vi "GetDistance2TL.vi"(3 "Traffic Lights":T1, 4 "Truck Dimensions":dbl[](array[numeric]), 5 "Trajectory Network":T2(array[cluster]), 6 "CurrentWP":i32[](array[numeric]), 7 "Trucks Poses":dbl[][](array[numeric]), 8 "Current State":i32[](array[numeric])=[1, 1, 1]) -> (0 "StopArray_2":i32[](array[numeric]), 1 "d2TLFinal":dbl[](array[numeric]), 2 "StopArray_1":i32[](array[numeric]))   [LabVIEW 2013]
uses:
  <vilib>/imath/engines/lvmath/Plug In/_Char/NIMS_CH_character datatype.ctl
  <vilib>/imath/engines/lvmath2/RunTimeEngine/ErrorHandling/NIMS_Finalize Error.vi
  <vilib>/imath/engines/lvmath2/RunTimeEngine/Managers/WorkSpace/UID Generator.vi
  <vilib>/imath/engines/lvmath2/RunTimeEngine/BuiltInFunctions/size/NIMS_I32=size(GM,I32).vi
  <instcachedir>/0/NIMS_I32=size(GM,I32)_0501686D1A7F4581B546512A0CE6115B.lvgen/NIMS_I32=size(GM,I32)_0501686D1A7F4581B546512A0CE6115B_004.vi
  <vilib>/imath/engines/lvmath2/RunTimeEngine/BuiltInFunctions/zeros/NIMS_M=zeros(I32,I32).vi
  <vilib>/imath/engines/lvmath2/RunTimeEngine/ErrorHandling/NIMS_Create Error From Enums.vi
  <vilib>/imath/engines/lvmath2/RunTimeEngine/BuiltInFunctions/ones/NIMS_M=ones(I32,I32).vi
  <vilib>/imath/engines/lvmath2/RunTimeEngine/BuiltInFunctions/zeros/NIMS_V=zeros(I32,I32).vi
  <vilib>/imath/engines/lvmath2/RunTimeEngine/RangeToken/NIMS_Range_R2 - Integer.vi
  <instcachedir>/0/NIMS_Range_R2 - Integer_C51C130E5EA5464EA148B28CDAB9615A.lvgen/NIMS_Range_R2 - Integer_C51C130E5EA5464EA148B28CDAB9615A_000.vi
  <vilib>/imathl/engines/lvmath/Functions/Error Handling/Create Error.vi
  <vilib>/imath/engines/lvmath2/RunTimeEngine/Managers/SymbolTable/Clear UID.vi
  <vilib>/imath/engines/lvmath2/RunTimeEngine/NodeEndStatement/NIMS_NodeEndStatement_Output.vi
  <instcachedir>/0/NIMS_NodeEndStatement_Output_53EC0D466D134D7ABD903AC30B43404B.lvgen/NIMS_NodeEndStatement_Output_53EC0D466D134D7ABD903AC30B43404B_004.vi
  <instcachedir>/0/NIMS_NodeEndStatement_Output_53EC0D466D134D7ABD903AC30B43404B.lvgen/NIMS_NodeEndStatement_Output_53EC0D466D134D7ABD903AC30B43404B_000.vi
  <vilib>/imath/engines/lvmath2/RunTimeEngine/CommandStatement/MC_CommandStatement_break.vi
  <vilib>/imath/engines/lvmath2/RunTimeEngine/IndexRead/NIMS V(S).vi
  <instcachedir>/0/NIMS V(S)_0488751826AF41519A22953C041130DC.lvgen/NIMS V(S)_0488751826AF41519A22953C041130DC_002.vi
  <vilib>/imath/engines/lvmath2/RunTimeEngine/IndexRead/NIMS M(S,S).vi
  <instcachedir>/0/NIMS M(S,S)_AC51E74150A542F7991B9634C66F3096.lvgen/NIMS M(S,S)_AC51E74150A542F7991B9634C66F3096_000.vi
  <vilib>/imath/engines/lvmath2/RunTimeEngine/BuiltInFunctions/deg_to_rad/NIMS_deg_to_rad.vi
  <instcachedir>/0/NIMS_deg_to_rad_4A81D684CE8D4DD79924F5AB74D756E1.lvgen/NIMS_deg_to_rad_4A81D684CE8D4DD79924F5AB74D756E1_001.vi
  <vilib>/imath/engines/lvmath2/RunTimeEngine/BuiltInFunctions/atan2/NIMS_atan2.vi
  <instcachedir>/0/NIMS_atan2_A91AA4A7D42247EDBE8F76DB99AF04A4.lvgen/NIMS_atan2_A91AA4A7D42247EDBE8F76DB99AF04A4_000.vi
  <vilib>/imath/engines/lvmath/Plug In/_Char/NIMS_CH_Character RV to String.vi
  <vilib>/imath/engines/lvmath2/RunTimeEngine/BuiltInFunctions/fprintf/NIMS_fprintf(Str,RS,RS).vi
  <vilib>/imath/engines/lvmath2/RunTimeEngine/IndexReplace/NIMS M(S,S)=S.vi
  <instcachedir>/0/NIMS M(S,S)=S_EC2A86BD47664E68AE45685B0A86CA9E.lvgen/NIMS M(S,S)=S_EC2A86BD47664E68AE45685B0A86CA9E_001.vi
  <vilib>/imath/engines/lvmath2/RunTimeEngine/RunTimeType/NIMS_RunTimeType_From StrictType (excl LVString).vi
  <instcachedir>/0/NIMS_RunTimeType_From StrictType (excl LVString)_4DEE718D6EB74582AA20236969C084FC.lvgen/NIMS_RunTimeType_From StrictType (excl LVString)_4DEE718D6EB74582AA20236969C084FC_000.vi
  <vilib>/imath/engines/lvmath2/RunTimeEngine/LocalVariableDefStatement/MC_LocalVariableDefStatement_Display.vi
  <vilib>/imath/engines/lvmath2/RunTimeEngine/IndexRead/NIMS M(S,$).vi
  <instcachedir>/0/NIMS M(S,$)_F24F360562DE41D8BE234322A2E15C65.lvgen/NIMS M(S,$)_F24F360562DE41D8BE234322A2E15C65_001.vi
  <vilib>/imath/engines/lvmath2/RunTimeEngine/BuiltInFunctions/sort/NIMS_sort(CRowV,I32,Str).vi
  <instcachedir>/0/NIMS_sort(CRowV,I32,Str)_29346373CFC04663A860DA4419001647.lvgen/NIMS_sort(CRowV,I32,Str)_29346373CFC04663A860DA4419001647_000.vi
  <vilib>/imath/engines/lvmath2/RunTimeEngine/BuiltInFunctions/findnz/NIMS_[1o]_findnz(GRowV).vi
  <instcachedir>/0/NIMS_[1o]_findnz(GRowV)_A907680C39E74AF18CBD76E991AC1137.lvgen/NIMS_[1o]_findnz(GRowV)_A907680C39E74AF18CBD76E991AC1137_000.vi
  <vilib>/imath/engines/lvmath2/RunTimeEngine/BuiltInFunctions/length/NIMS_length(GV).vi
  <instcachedir>/0/NIMS_length(GV)_08A3D13377FD4E4B96F5795FBF3698FA.lvgen/NIMS_length(GV)_08A3D13377FD4E4B96F5795FBF3698FA_002.vi
  <vilib>/imath/engines/lvmath2/RunTimeEngine/VariableToken/Support/NIMS_Vector Boolean Index to I32 Index.vi
  <vilib>/imath/engines/lvmath2/RunTimeEngine/IndexReplace/NIMS V(V)=M.vi
  <instcachedir>/0/NIMS V(V)=M_3D179AF5652E4922BC7E7B3B6BD740B2.lvgen/NIMS V(V)=M_3D179AF5652E4922BC7E7B3B6BD740B2_000.vi
  <instcachedir>/0/NIMS V(S)_0488751826AF41519A22953C041130DC.lvgen/NIMS V(S)_0488751826AF41519A22953C041130DC_005.vi
  <vilib>/imath/engines/lvmath2/RunTimeEngine/IndexReplace/NIMS V(S)=S.vi
  <instcachedir>/0/NIMS V(S)=S_66A18068148B4981A312229A93EA5C06.lvgen/NIMS V(S)=S_66A18068148B4981A312229A93EA5C06_001.vi
  <vilib>/imath/engines/lvmath2/RunTimeEngine/IndexRead/NIMS V(R2).vi
  <instcachedir>/0/NIMS V(R2)_C76619605A0E4E9F8B2FA9389712AC47.lvgen/NIMS V(R2)_C76619605A0E4E9F8B2FA9389712AC47_002.vi
  <vilib>/imath/engines/lvmath2/RunTimeEngine/IndexRead/NIMS V(V).vi
  <instcachedir>/0/NIMS V(V)_298D9CB7BFEB42B8BC8D9C3C28AE8C70.lvgen/NIMS V(V)_298D9CB7BFEB42B8BC8D9C3C28AE8C70_002.vi
  <vilib>/imath/engines/lvmath2/RunTimeEngine/BuiltInFunctions/sum/NIMS_sum(GV).vi
  <instcachedir>/0/NIMS_sum(GV)_67F5EC36BC034E54A6BEC5B0673C00E5.lvgen/NIMS_sum(GV)_67F5EC36BC034E54A6BEC5B0673C00E5_000.vi
  <vilib>/imath/engines/lvmath2/RunTimeEngine/Managers/SymbolTable/NIMS_WorkSpace.lvlib
panel:
  out "StopArray_2_before":i32[](array[numeric])
  out "d2TL_1":dbl[](array[numeric])
  out "d2TL_2":dbl[](array[numeric])
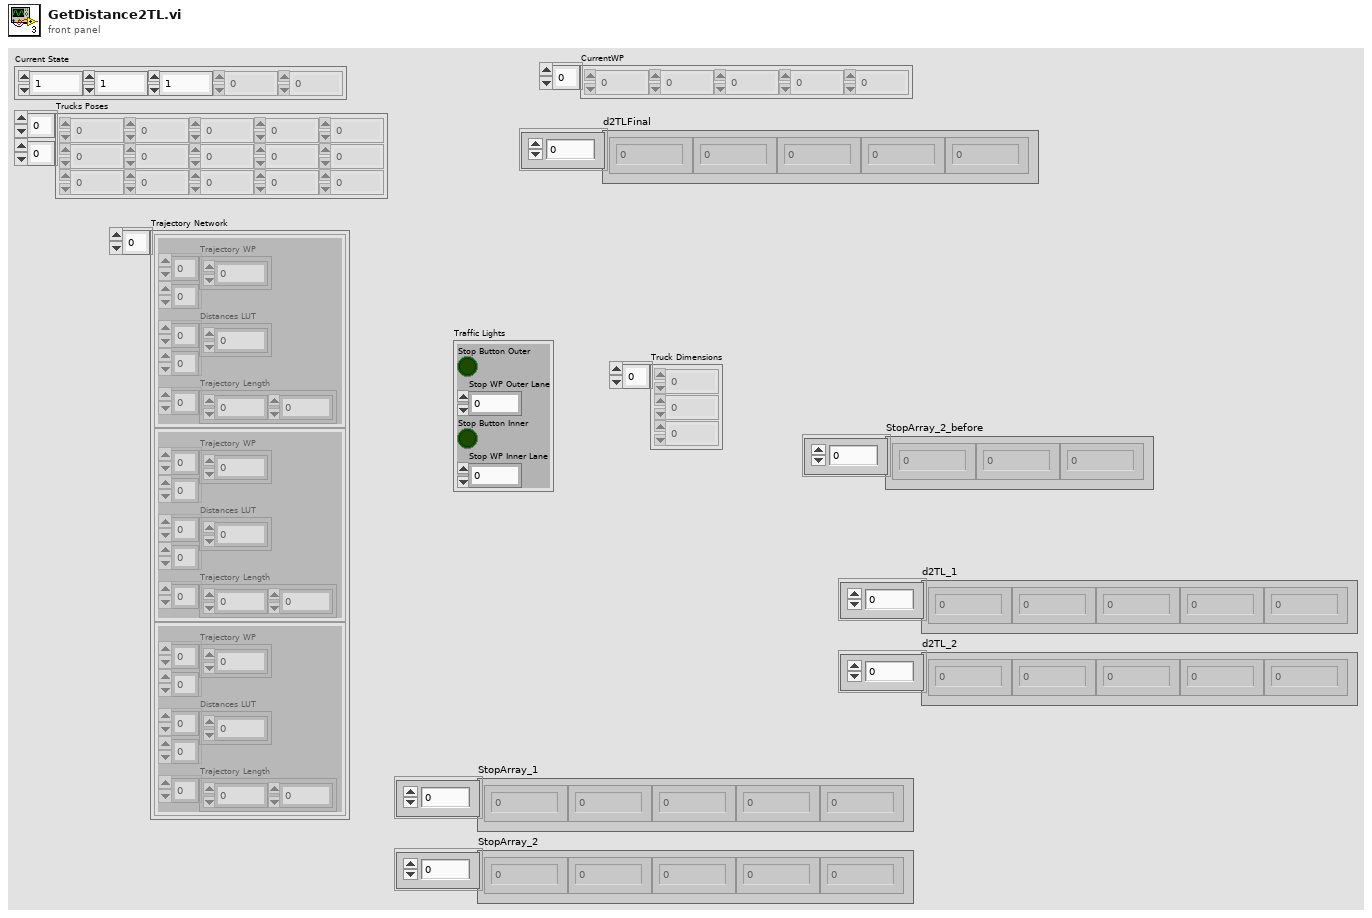
[diagram p1: front panel]
types:
  T1 = cluster{"Stop Button Outer":bool, "Stop WP Outer Lane":i32, "Stop Button Inner":bool, "Stop WP Inner Lane ":i32}
  T2 = cluster{"Trajectory WP":dbl[][], "Distances LUT":dbl[][], "Trajectory Length":i32[]}[]
  T3 = cluster{"Trajectory WP":dbl[][], "Distances LUT":dbl[][], "Trajectory Length":i32[]}
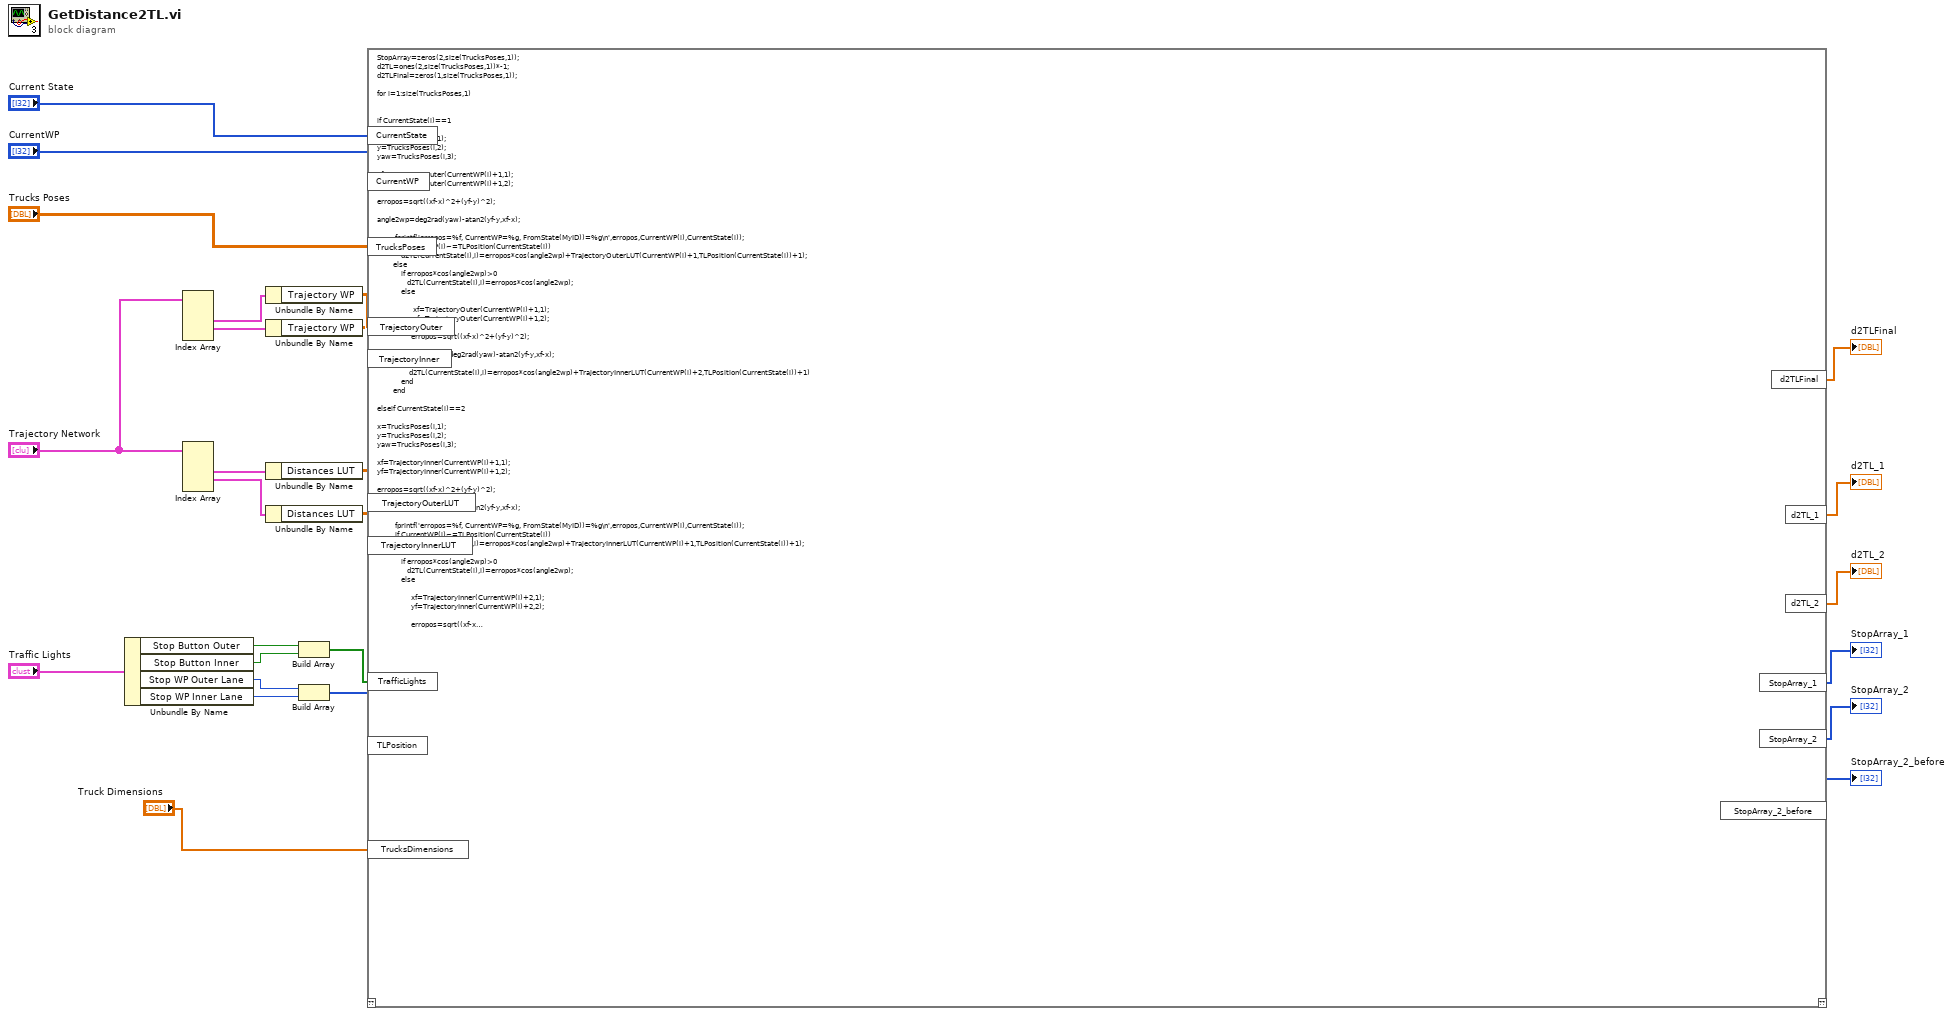
[diagram p0: block diagram]
diagram:
  n1 = Unbundle By Name("Traffic Lights") -> ("Stop Button Outer"=w15:bool, "Stop Button Inner"=w14:bool, "Stop WP Outer Lane"=w12:i32, "Stop WP Inner Lane"=w13:i32)
  n2 = Index Array(array="Trajectory Network") -> (element #2=w24:T3, element #3=w25:T3)  [unwired: 4 in, 2 out]
  n3 = Index Array(array="Trajectory Network") -> (element #2=w21:T3, element #3=w20:T3)  [unwired: 4 in, 2 out]
  n4 = Unbundle By Name(w24) -> ("Trajectory WP"=w23:dbl[][])
  n5 = Unbundle By Name(w25) -> ("Trajectory WP"=w22:dbl[][])
  n6 = Unbundle By Name(w21) -> ("Distances LUT"=w18:dbl[][])
  n7 = Unbundle By Name(w20) -> ("Distances LUT"=w17:dbl[][])
  n8 = Build Array(w15, w14) -> (w11:bool[])
  n9 = Build Array(w12, w13) -> (w10:i32[])
  n10 = mathscript code="StopArray=zeros(2,size(TrucksPoses,1));\nd2TL=ones(2,size(TrucksPoses,1))*-1;\nd2TLFinal=zeros(1,size(TrucksPoses,1));\n\nfor i=1:size(TrucksPoses,1)\n\n\nif CurrentState(i)==1\n\nx=TrucksPoses(i,1);\ny=TrucksPoses(i,2);\nyaw=TrucksPoses(i,3);\n\nxf=TrajectoryOuter(CurrentWP(i)+1,1);\nyf=TrajectoryOuter(CurrentWP(i)+1,2);\n\nerropos=sqrt((xf-x)^2+(yf-y)^2);\n\nangle2wp=deg2rad(yaw)-atan2(yf-y,xf-x);\n\n         fprintf('erropos=%f, CurrentWP=%g, FromState(MyID))=%g\\n',erropos,CurrentWP(i),CurrentState(i));\n         if CurrentWP(i)~=TLPosition(CurrentState(i))\n            d2TL(CurrentState(i),i)=erropos*cos(angle2wp)+TrajectoryOuterLUT(CurrentWP(i)+1,TLPosition(CurrentState(i))+1);\n        else\n            if erropos*cos(angle2wp)>0\n               d2TL(CurrentState(i),i)=erropos*cos(angle2wp);\n            else\n\n                  xf=TrajectoryOuter(CurrentWP(i)+1,1);\n                  yf=TrajectoryOuter(CurrentWP(i)+1,2);\n\n                 erropos=sqrt((xf-x)^2+(yf-y)^2);\n\n                 angle2wp=deg2rad(yaw)-atan2(yf-y,xf-x);\n                \n                d2TL(CurrentState(i),i)=erropos*cos(angle2wp)+TrajectoryInnerLUT(CurrentWP(i)+2,TLPosition(CurrentState(i))+1)\n            end\n        end\n\nelseif CurrentState(i)==2\n\nx=TrucksPoses(i,1);\ny=TrucksPoses(i,2);\nyaw=TrucksPoses(i,3);\n\nxf=TrajectoryInner(CurrentWP(i)+1,1);\nyf=TrajectoryInner(CurrentWP(i)+1,2);\n\nerropos=sqrt((xf-x)^2+(yf-y)^2);\n\nangle2wp=deg2rad(yaw)-atan2(yf-y,xf-x);\n\n         fprintf('erropos=%f, CurrentWP=%g, FromState(MyID))=%g\\n',erropos,CurrentWP(i),CurrentState(i));\n         if CurrentWP(i)~=TLPosition(CurrentState(i))\n            d2TL(CurrentState(i),i)=erropos*cos(angle2wp)+TrajectoryInnerLUT(CurrentWP(i)+1,TLPosition(CurrentState(i))+1);\n        else\n            if erropos*cos(angle2wp)>0\n               d2TL(CurrentState(i),i)=erropos*cos(angle2wp);\n            else\n\n                 xf=TrajectoryInner(CurrentWP(i)+2,1);\n                 yf=TrajectoryInner(CurrentWP(i)+2,2);\n\n                 erropos=sqrt((xf-x)^2+(yf-y)^2);\n\n                 angle2wp=deg2rad(yaw)-atan2(yf-y,xf-x);\n                \n                d2TL(CurrentState(i),i)=erropos*cos(angle2wp)+TrajectoryInnerLUT(CurrentWP(i)+2,TLPosition(CurrentState(i))+1)\n            end\n        end\n\nend\n\nend\n\nd2TL_1=d2TL(1,:);\nd2TL_2=d2TL(2,:);\n\n\n[spare, StopArray_1]=sort(d2TL_1);\n[spare, StopArray_2]=sort(d2TL_2);\n\nStopArray_2_before=StopArray_2;\n\nf1=find(d2TL_1==-1);\nf2=find(d2TL_2==-1)\n\nif length(f1)>0\n    for i=1:length(f1)\n        StopArray_1(StopArray_1==f1(i))=[];\n    end\nend\nif length(f2)>0\n    for i=1:length(f2)\n        StopArray_2(StopArray_2==f2(i))=[];\n    end\nend\n\ndref2TL=0.3;\n\nif length(StopArray_1)>0\n    d2TLFinal(StopArray_1(1))=d2TL_1(StopArray_1(1));\n    for i=2:length(StopArray_1)\n        d2TLFinal(StopArray_1(i))=d2TL_1(StopArray_1(i))-sum(TrucksDimensions(StopArray_1(1:i-1)))-dref2TL*(i-1);\n    end\nend\n\nif length(StopArray_2)>0\n    d2TLFinal(StopArray_2(1))=d2TL_2(StopArray_2(1));\n    for i=2:length(StopArray_2)\n        d2TLFinal(StopArray_2(i))=d2TL_2(StopArray_2(i))-sum(TrucksDimensions(StopArray_2(1:i-1)))-dref2TL*(i-1);\n    end\nend\n\nStopArray_1=[StopArray_1,zeros(1,size(TrucksPoses,1)-length(StopArray_1))];\nStopArray_2=[StopArray_2,zeros(1,size(TrucksPoses,1)-length(StopArray_2))];"("CurrentState"="Current State", "CurrentWP"="CurrentWP", "TrucksPoses"="Trucks Poses", "TrafficLights"=w11, "TrajectoryOuterLUT"=w18, "TLPosition"=w10, "TrajectoryInner"=w22, "TrajectoryOuter"=w23, "TrajectoryInnerLUT"=w17, "TrucksDimensions"="Truck Dimensions") -> ("d2TLFinal"=→"d2TLFinal":cdb[], "d2TL_1"=→"d2TL_1":cdb[], "d2TL_2"=→"d2TL_2":cdb[], "StopArray_1"=→"StopArray_1":i32[], "StopArray_2"=→"StopArray_2":i32[], "StopArray_2_before"=→"StopArray_2_before":i32[])  [unwired: 1 in, 1 out]
